vi "Main.vi"() -> ()   [LabVIEW 2017]
doc: "The myRIO Project template acquires acceleration data from the onboard accelerometer and displays the changes of acceleration values in a waveform chart."
uses:
  <vilib>/userdefined/High Color/IMAQdx.ctl
  <vilib>/Platform/TimedLoop/XDataNode/timing_clust.ctl
  <vilib>/Platform/TimedLoop/XDataNode/nitl_modes.ctl
  <vilib>/Platform/TimedLoop/XDataNode/wakeup.ctl
  <vilib>/myRIO/Common/Instrument Driver Framework/myRIO v1.0/UART/vis/myRIO v1.0 Close UART.vi
  Global 1.vi
  Outputs.vi
  Inputs.vi
  <vilib>/myRIO/Common/Instrument Driver Framework/Utilities/vis/FPGA Ref Manager.vi
  <vilib>/myRIO/Common/Instrument Driver Framework/myRIO v1.0/myRIO v1.0 Reset FPGA.vi
  <vilib>/myRIO/Common/Instrument Driver Framework/myRIO v1.0/IRQ/vis/myRIO v1.0 IRQ Info FGV.vi
  <vilib>/myRIO/Common/Instrument Driver Framework/myRIO v1.0/IRQ/vis/myRIO v1.0 Timer IRQ Info FGV.vi
  <vilib>/myRIO/Common/Instrument Driver Framework/myRIO v1.0/IRQ/vis/myRIO v1.0 ISR Agent.vi
  <vilib>/platform/TimedLoop/XDataNode/XDataNode.xnode
  <vilib>/Platform/TimedLoop/XDataNode/XDNodeRunTimeDep.lvlib
  <vilib>/myRIO/Instrument Drivers/Utilities/Utilities.lvlib
  <vilib>/vision/driver/NI_Vision_Acquisition_Software.lvlib
panel:
  out "Step":i16
  in  "Start":bool
  out "error out":errorcluster
  in  "Stop":bool
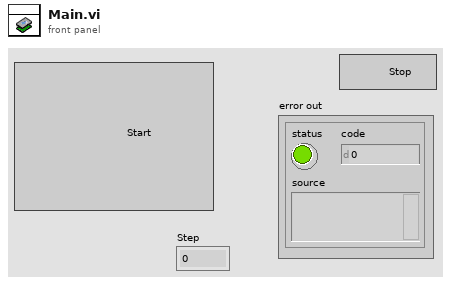
[diagram p1: front panel]
types:
  T1 = typedef "IMAQdx.ctl" = refnum<k21>
  T2 = typedef "XDNodeRunTimeDep.lvlib/timing_clust.ctl" = cluster{"Expected End [f-1]":u64, "Actual End [f-1]":u64, "Finished Late? [f-1]":bool, "Expected End [i-1]":u64, "Actual End [i-1]":u64, "Finished Late? [i-1]":bool, "Expected Start [i]":u64, "Actual Start [i]":u64, "Expected Start [f]":u64, "Actual Start [f]":u64, "Source Name":string, "Structure Name":string, "Period":i64, "Deadline":i64, "Offset":i64, "Start":i64, "Priority":i32, "Timeout":i32, "Mode":T3, "Wakeup Reason":T4, "Error":errorcluster, "Source Type":string, "Secondary Source Type":string, "Global End Time":u64, "Global Start Time":u64, "Frame Duration":u64, "Iteration Duration":u64, "Assigned CPU":i32, "I/O Scan Engine Mode":u32}
  T3 = typedef "XDNodeRunTimeDep.lvlib/nitl_modes.ctl" = enum32{"No Change", "Process missed periods, maintain original phase", "Discard missed periods, maintain original phase", "Process missed periods, ignore original phase", "Discard missed periods, ignore original phase"}
  T4 = typedef "XDNodeRunTimeDep.lvlib/wakeup.ctl" = enum32{"Normal", "Aborted", "Asynchronous wakeup", "Timing source error", "Timed loop error", "Timeout"}
  T5 = typedef "I2C.lvlib/I2C Reference.ctl" = cluster{"myRIO Reference":T6, "I2C Channels Enum":T10, "I2C Configuration":T11}
  T6 = typedef "myRIO Generic Hardware Reference.ctl" = cluster{"myRIO Model":T7, "myRIO Hardware Reference":T8}
  T7 = typedef "Hardware Version Enum.ctl" = enum16{"Unknown", "myRIO-1900", "myRIO-1950", "roboRIO", "NI ELVIS RIO CM"}
  T8 = typedef "myRIO v1.0 Reference.ctl" = cluster{"Generic FPGA Reference":T9, "Allow multiple opens":bool}
  T9 = typedef "Generic FPGA Reference.ctl" = refnum<k20>
  T10 = typedef "I2C Channels Enum.ctl" = enum16{"Not Connected", "A/I2C", "B/I2C", "I2C/I2C"}
  T11 = typedef "I2C.lvlib/I2C Configuration.ctl" = cluster{"I2C Transfer Rate":T12}
  T12 = typedef "I2C.lvlib/I2C Transfer Rate.ctl" = enum16{"Standard mode (100 kbps)", "Fast mode (400 kbps)"}
  T13 = typedef "IMAQ Image.ctl" = refnum<image>
  T14 = typedef "IMAQ GM Match Report.ctl" = cluster{"Position":cluster{"x":sgl, "y":sgl}, "Angle":sgl, "Scale":sgl, "Score":sgl, "Bounding Box":cluster{"x":sgl, "y":sgl}[], "Contrast Reversed":bool, "Occlusion %":sgl, "Template Target Curve Score":sgl, "Target Template Curve Score":sgl, "Correlation Score":sgl}
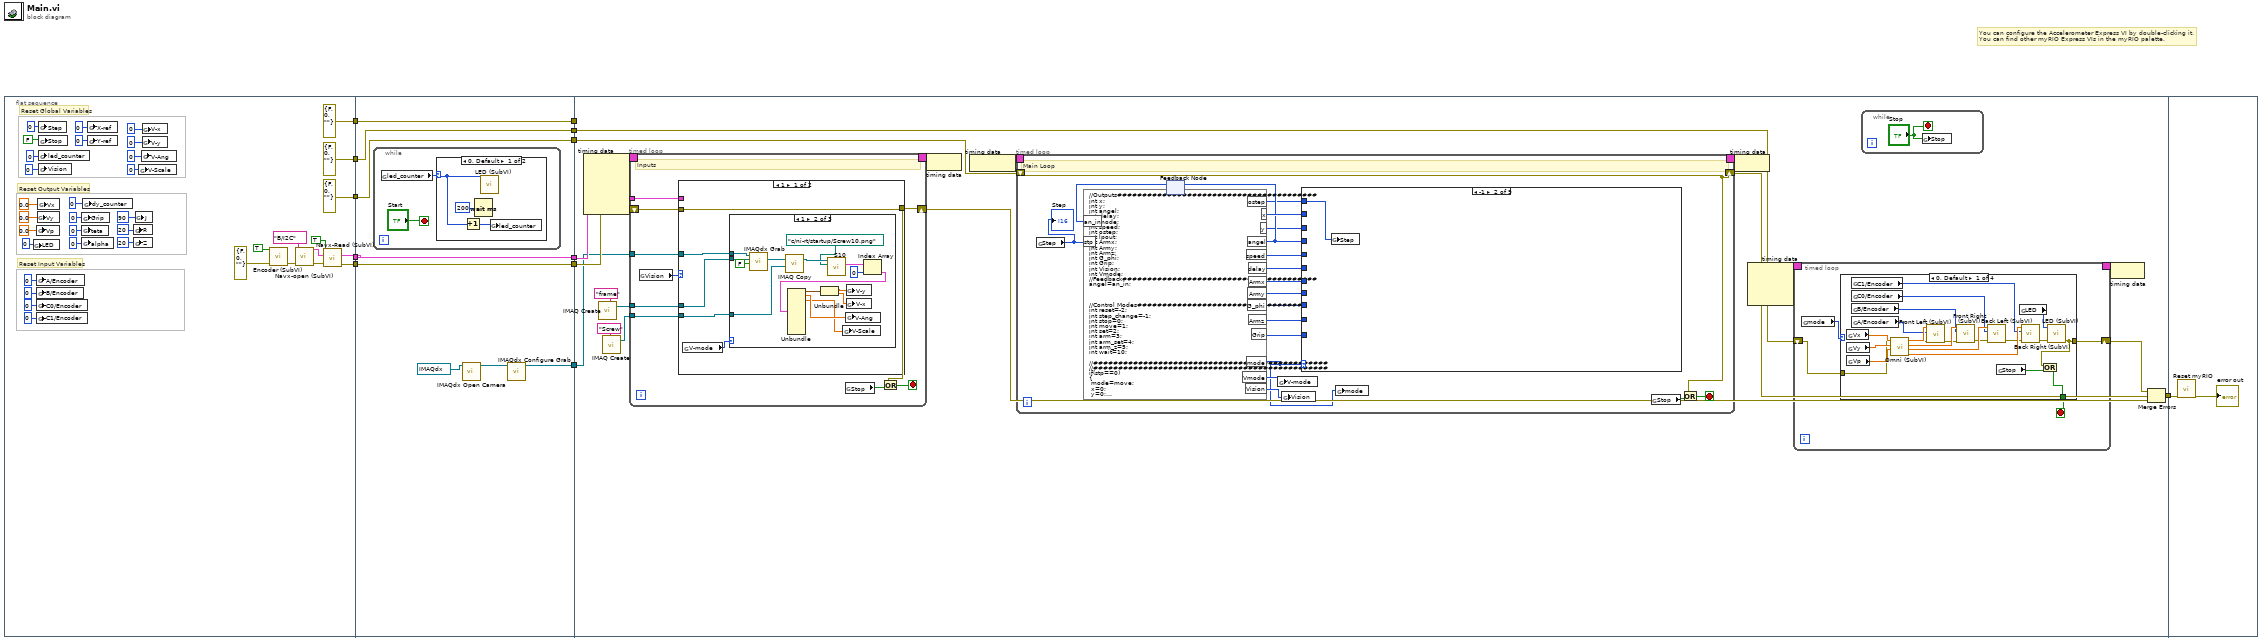
[diagram p0: block diagram]
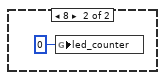
[diagram p2: hidden frame]
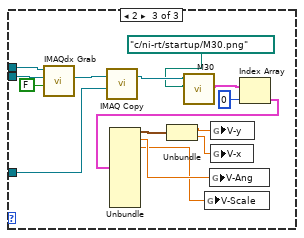
[diagram p4: hidden frame]
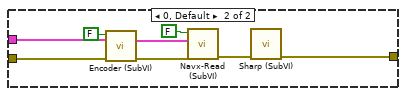
[diagram p5: hidden frame]
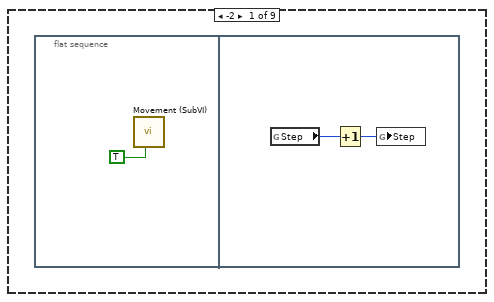
[diagram p6: hidden frame]
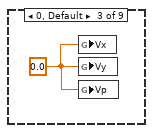
[diagram p7: hidden frame]
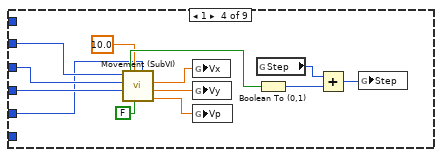
[diagram p8: hidden frame]
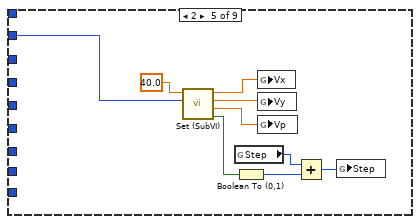
[diagram p9: hidden frame]
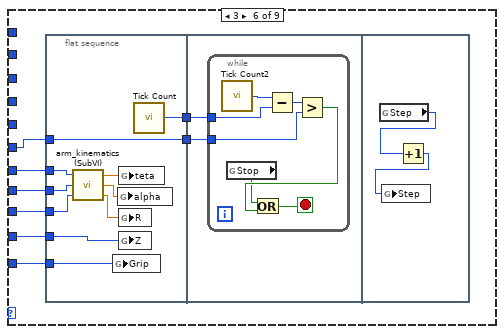
[diagram p10: hidden frame]
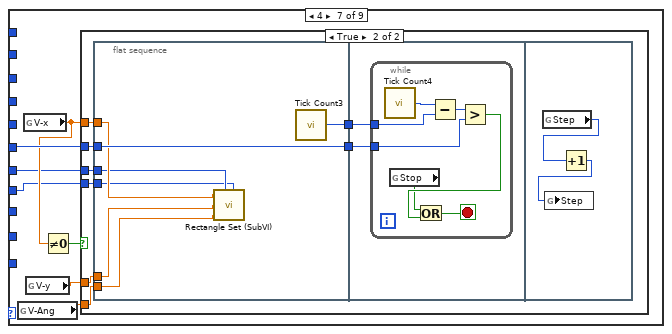
[diagram p11: hidden frame]
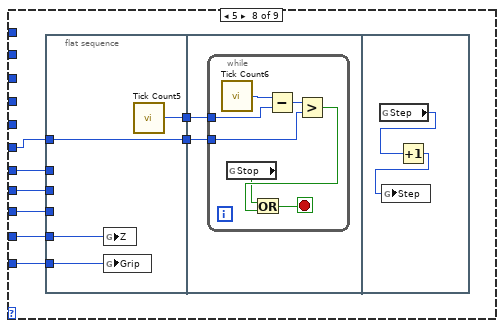
[diagram p13: hidden frame]
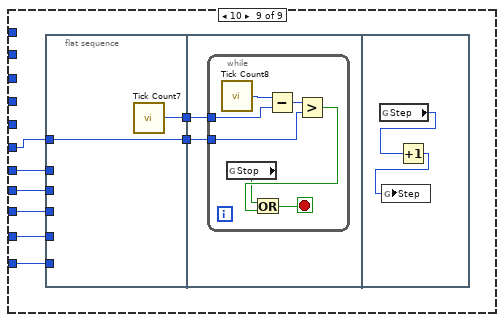
[diagram p14: hidden frame]
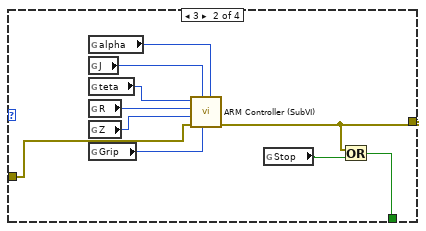
[diagram p15: hidden frame]
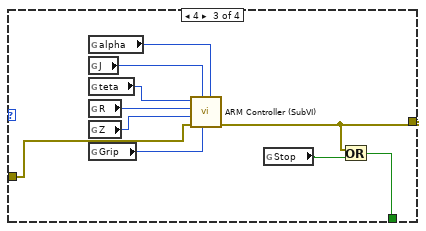
[diagram p16: hidden frame]
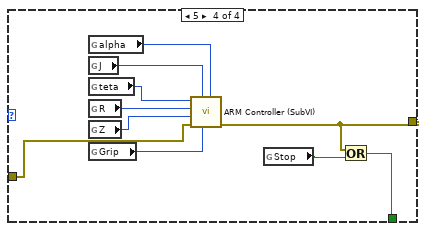
[diagram p17: hidden frame]
diagram:
  # "You can configure the Accelerometer Express VI by double-clicking it.\nYou can find other myRIO Express VIs in the myRIO palette."
  n1 = flat-sequence {
    tunnel: [w44] -> w12
    tunnel: [errorcluster {"status"=FALSE, "code"=0, "source"=""} ("error in (no error)")] -> w10
    tunnel: [errorcluster {"status"=FALSE, "code"=0, "source"=""} ("error in (no error)")] -> w8
    tunnel: [w42] -> w7
    tunnel: [errorcluster {"status"=FALSE, "code"=0, "source"=""} ("error in (no error)")] -> w4
    tunnel: w12 -> [w56]
    tunnel: [w56] -> w11
    tunnel: w10 -> [w55]
    tunnel: [w55] -> w9
    tunnel: w8 -> [w52]
    tunnel: w7 -> [w54]
    tunnel: [w54] -> w6
    tunnel: [w53] -> w5
    tunnel: w4 -> [w53]
    tunnel: [w52] -> w2
    tunnel: [w49] -> w1
    tunnel: w11 -> [w81]
    tunnel: w9 -> [_]
    tunnel: w6 -> [w74]
    tunnel: w5 -> [w73]
    tunnel: [w72] -> w3
    tunnel: w2 -> [w68]
    tunnel: w1 -> [w67]
    tunnel: w3 -> [w352]
    frame #0 {
      # "Reset Global Variables"
      # "Reset Input Variables"
      # "Reset Output Variables"
      # "Initialize"
      n2 = global write "Outputs.vi" "LED"(i8 0 ("LED")) -> ()
      n3 = global write "Outputs.vi" "Vp"(0.0 ("Vp")) -> ()
      n4 = global write "Inputs.vi" "A/Encoder"(0 ("A/Encoder")) -> ()
      n5 = global write "Inputs.vi" "B/Encoder"(0 ("B/Encoder")) -> ()
      n6 = global write "Inputs.vi" "C0/Encoder"(0 ("C0/Encoder")) -> ()
      n7 = global write "Inputs.vi" "C1/Encoder"(0 ("C1/Encoder")) -> ()
      n8 = global write "Outputs.vi" "Vy"(0.0 ("Vy")) -> ()
      n9 = global write "Outputs.vi" "Vx"(0.0 ("Vx")) -> ()
      n10 = global write "Global 1.vi" "Step"(i16 0 ("Step")) -> ()
      n11 = global write "Global 1.vi" "led_counter"(i8 0 ("Step")) -> ()
      n12 = global write "Global 1.vi" "Vision"(i8 0 ("Step")) -> ()
      n13 = global write "Global 1.vi" "Stop"(FALSE ("Stop")) -> ()
      n14 = global write "Outputs.vi" "Grip"(i16 0 ("Grip")) -> ()
      n15 = global write "Outputs.vi" "teta"(i16 0 ("teta")) -> ()
      n16 = global write "Outputs.vi" "alpha"(i16 0 ("alpha")) -> ()
      n17 = global write "Outputs.vi" "dy_counter"(i8 0 ("LED")) -> ()
      n18 = global write "Global 1.vi" "X-ref"(i64 0 ("X-ref")) -> ()
      n19 = global write "Global 1.vi" "Y-ref"(i64 0 ("Y-ref")) -> ()
      n20 = global write "Outputs.vi" "R"(i16 20 ("R")) -> ()
      n21 = global write "Outputs.vi" "Z"(i16 20 ("Z")) -> ()
      n22 = global write "Outputs.vi" "J"(i16 90 ("J")) -> ()
      n23 = global write "Global 1.vi" "V-Scale"(i64 0 ("Y-ref")) -> ()
      n24 = global write "Global 1.vi" "V-Ang"(i64 0 ("X-ref")) -> ()
      n25 = global write "Global 1.vi" "V-x"(i64 0 ("X-ref")) -> ()
      n26 = global write "Global 1.vi" "V-y"(i64 0 ("Y-ref")) -> ()
      n27 = call "Encoder (SubVI).vi"("error in (no error)"=errorcluster {"status"=FALSE, "code"=0, "source"=""}, "Reset?"=TRUE ("Reset Counter")) -> ("error out"=w26:errorcluster)  [unwired: 9 in]
      n28 = call "Navx-open (SubVI).vi"("error in (no error)"=w26, "Channel Name"=tag "B/I2C") -> ("error out"=w46:errorcluster, "I2C Ref Out"=w42:T5)  [unwired: 8 in]
      n29 = call "Navx-Read (SubVI).vi"("error in (no error)"=w46, "I2C Ref Out"=w42, "Reset"=TRUE) -> ("error out"=w44:errorcluster)  [unwired: 7 in, 1 out]
    }
    frame #1 {
      n30 = while {
        stop <- "Start" stop-if-true
        n31 = global read "Global 1.vi" "led_counter"() -> (w57:i8)
        n32 = case shown="0, Default" w57 {
          selector: w57 -> [w59 _]
          frame 0, Default {
            n33 = Increment(x=w59) -> (x+1=w61:i8)
            n34 = Wait (ms)(milliseconds to wait=u32 200) -> ()  [unwired: 1 out]
            n35 = call "LED (SubVI).vi"("LED"=w59) -> ()  [unwired: 10 in, 1 out]
            n36 = global write "Global 1.vi" "led_counter"(w61) -> ()
          }
          frame 8 {
            n37 = global write "Global 1.vi" "led_counter"(i8 0 ("led_counter")) -> ()
          }
        }
      }
      n38 = call <vilib>:"IMAQdx Open Camera.vi"("Session In"=T1 "cam0") -> ("Session Out"=w50:T1)  [unwired: 9 in, 1 out]
      n39 = call <vilib>:"IMAQdx Configure Grab.vi"("Session In"=w50) -> ("Session Out"=w49:T1)  [unwired: 9 in, 1 out]
    }
    frame #2 {
      n40 = node-c288() -> (w76:T2)  [unwired: 5 in]
      n41 = call "IMAQ Create"("Image Name"="frame") -> ("New Image"=w64:T13)  [unwired: 4 in, 1 out]
      n42 = call "IMAQ Create"("Image Name"="Screw") -> ("New Image"=w63:T13)  [unwired: 4 in, 1 out]
      n43 = timed-loop {
        shift-right: [w86] -> w71
        shift-left: w81 -> [w90]
        timing: w76 -> [_]
        timing-out: [_] -> w75
        tunnel: w74 -> [w88]
        tunnel: w67 -> [w84]
        tunnel: w64 -> [w83]
        tunnel: w63 -> [w82]
        stop <- w89 stop-if-true
        # "Inputs"
        n44 = global read "Global 1.vi" "Vision"() -> (w85:i16)
        n45 = case shown="1" w85 {
          tunnel: w90 -> [w92 w132]
          tunnel: w88 -> [_ w129]
          tunnel: [w92 w127] -> w86
          tunnel: w84 -> [w95 _]
          tunnel: w83 -> [w94 _]
          tunnel: w82 -> [w93 _]
          frame 1 {
            n46 = global read "Global 1.vi" "V-mode"() -> (w91:i16)
            n47 = case shown="1" w91 {
              tunnel: w94 -> [_ w108 w124]
              tunnel: w93 -> [_ w107 w123]
              tunnel: w95 -> [_ w97 w115]
              frame 0, Default {
              }
              frame 1 {
                n48 = call <vilib>:"IMAQdx Grab.vi"("Wait for Next Buffer? (Yes)"=FALSE, "Image In"=w108, "Session In"=w97) -> ("Image Out"=w110:T13)  [unwired: 5 in, 3 out]
                n49 = call "IMAQ Copy"("Image Dst"=w107, "Image Src"=w110) -> ("Image Dst Out"=w109:T13)  [unwired: 4 in, 1 out]
                n50 = call "S10.vi"("Template File Path (Geometric Matching 1)"=path "c:/ni-rt/startup/Screw10.png", "Image In"=w109) -> ("Matches (Geometric Matching 1)"=w105:T14[])  [unwired: 5 in, 2 out]
                n51 = Index Array(array=w105, index=0) -> (element=w103:T14)
                n52 = Unbundle(w103) -> ("Position"=w102:cluster{"x":sgl, "y":sgl}, "Angle"=w99:sgl, "Scale"=w98:sgl)  [unwired: 7 out]
                n53 = Unbundle(w102) -> ("x"=w101:sgl, "y"=w100:sgl)
                n54 = global write "Global 1.vi" "V-Scale"(w98) -> ()
                n55 = global write "Global 1.vi" "V-Ang"(w99) -> ()
                n56 = global write "Global 1.vi" "V-y"(w101) -> ()
                n57 = global write "Global 1.vi" "V-x"(w100) -> ()
              }
              frame 2 {
                n58 = call <vilib>:"IMAQdx Grab.vi"("Wait for Next Buffer? (Yes)"=FALSE, "Image In"=w124, "Session In"=w115) -> ("Image Out"=w125:T13)  [unwired: 5 in, 3 out]
                n59 = call "IMAQ Copy"("Image Dst"=w123, "Image Src"=w125) -> ("Image Dst Out"=w113:T13)  [unwired: 4 in, 1 out]
                n60 = call "M30.vi"("Template File Path (Geometric Matching 1)"=path "c:/ni-rt/startup/M30.png", "Image In"=w113) -> ("Matches (Geometric Matching 1)"=w114:T14[])  [unwired: 3 in, 2 out]
                n61 = Index Array(array=w114, index=0) -> (element=w121:T14)
                n62 = Unbundle(w121) -> ("Position"=w120:cluster{"x":sgl, "y":sgl}, "Angle"=w117:sgl, "Scale"=w116:sgl)  [unwired: 7 out]
                n63 = Unbundle(w120) -> ("x"=w119:sgl, "y"=w118:sgl)
                n64 = global write "Global 1.vi" "V-Scale"(w116) -> ()
                n65 = global write "Global 1.vi" "V-Ang"(w117) -> ()
                n66 = global write "Global 1.vi" "V-y"(w119) -> ()
                n67 = global write "Global 1.vi" "V-x"(w118) -> ()
              }
            }
          }
          frame 0, Default {
            n68 = call "Encoder (SubVI).vi"("error in (no error)"=w132, "Reset?"=FALSE ("Boolean")) -> ("error out"=w130:errorcluster)  [unwired: 9 in]
            n69 = call "Navx-Read (SubVI).vi"("error in (no error)"=w130, "I2C Ref Out"=w129, "Reset"=FALSE) -> ("error out"=w128:errorcluster)  [unwired: 7 in, 1 out]
            n70 = call "Sharp (SubVI).vi"("error in (no error)"=w128) -> ("error out"=w127:errorcluster)  [unwired: 10 in]
          }
        }
        n71 = global read "Global 1.vi" "Stop"() -> (w87:bool)
        n72 = Or(x=w86, y=w87) -> (x .or. y?=w89:bool)
      }
      n73 = node-c288(w75) -> ()
      n74 = node-c288() -> (w78:T2)
      n75 = timed-loop {
        shift-right: [w154] -> w70
        shift-left: w68 -> [w154]
        timing: w78 -> [_]
        timing-out: [_] -> w77
        stop <- w155 stop-if-true
        # "Main Loop"
        n76 = global read "Global 1.vi" "Step"() -> (w147:i16)
        "Step" <- w147
        n77 = feedback #1() -> (w151:i32)  [unwired: 1 in]
        n78 = formula code="//Outputs########################################\nint x;\nint y;\nint angel;\nint delay;\nint mode;\nint speed;\nint ostep;\nint lpout;\nint Armx;\nint Army;\nint Armz;\nint G_phi;\nint Grip;\nint Vision;\nint Vmode;\n//Feedback#######################################\nangel=an_in;\n\n\n\n//Control Modes##################################\nint reset=-2;\nint step_change=-1; \nint stop=0;\nint move=1;\nint set=2;\nint arm=3;\nint arm_set=4;\nint arm_z=5;\nint wait=10;\n\n//###############################################\n//###############################################\nif(stp==0)\n{\n\tmode=move;\n\tx=0;\n\ty=0;\n\tangel=0;\n\tspeed=50;\n}\nif(stp==1)\n{\n\tmode=arm;\n\tArmx=75;\n\tArmy=0;\n\tArmz=180;\n\tdelay=4000;\n\t\n}\nif(stp==2)\n{\n\tmode=step_change;\n\tostep=5;\n}\nif(stp==3)\n{\n\tmode=move;\n\tx=0;\n\ty=0;\n\tangel=-90;\n\tspeed=80;\n}\nif(stp==4)\n{\n\tmode=move;\n\tx=800;\n\ty=0;\n\tangel=0;\n\tspeed=80;\n}\nif(stp==5)\n{\n\tmode=set;\n\tx=3;\n\tspeed=50;\n}\nif(stp==6)\n{\n\tmode=reset;\n}\n\nif(stp==7)\n{\n\tmode=arm;\n\tArmx=75;\n\tArmy=0;\n\tArmz=280;\n\tdelay=4000;\n}\nif(stp==8)\n{\n\tVision=1;\n\tVmode=1;\n\tmode=wait;\n\tdelay=1500;\n}\nif(stp==9)\n{\n\tVision=1;\n\tVmode=1;\n\tmode=arm_set;\n\tArmx=75;\n\tArmy=0;\n\tdelay=4000;\n}\nif(stp==10)\n{\n\tVision=0;\n\tmode=wait;\n\tdelay=1000;\n}\nif(stp==11)\n{\n\tVision=0;\n\tmode=arm_z;\n\tArmz=100;\n\tGrip=0;\n\tdelay=3000;\n}\nif(stp==12)\n{\n\tmode=arm_z;\n\tArmz=100;\n\tGrip=1;\n\tdelay=1000;\n}\nif(stp==13)\n{\n\tmode=arm_z;\n\tArmz=200;\n\tGrip=1;\n\tdelay=1000;\n}\nif(stp==14)\n{\n\tmode=arm;\n\tArmx=75;\n\tArmy=0;\n\tArmz=200;\n\tGrip=1;\n\tdelay=4000;\n}\n\n\n\nif(stp==15)\n{\n\tmode=stop;\n}"("stp"=w147, "an_in"=w151) -> ("x"=w153:i32, "y"=w148:i32, "mode"=w137:i32, "angel"=w150:i32, "delay"=w152:i32, "speed"=w149:i32, "ostep"=w145:i32, "Armx"=w143:i32, "Army"=w142:i32, "Armz"=w141:i32, "G_phi"=w144:i32, "Grip"=w140:i32, "Vision"=w139:i32, "Vmode"=w138:i32)
        n79 = feedback-in #1(w150) -> ()
        n80 = global write "Global 1.vi" "V-mode"(w138) -> ()
        n81 = global write "Global 1.vi" "Vision"(w139) -> ()
        n82 = case shown="-1" w137 {
          tunnel: w153 -> [_ _ _ w167 w182 _ _ _ _]
          tunnel: w148 -> [_ _ _ w166 _ _ _ _ _]
          tunnel: w150 -> [_ _ _ w165 _ _ _ _ _]
          tunnel: w152 -> [_ _ _ _ _ w189 w218 w251 w274]
          tunnel: w149 -> [_ _ _ w164 _ _ _ _ _]
          tunnel: w145 -> [_ w159 _ _ _ _ _ _ _]
          tunnel: w144 -> [_ _ _ _ _ w185 _ w247 w270]
          tunnel: w143 -> [_ _ _ _ _ w187 w213 w249 w272]
          tunnel: w142 -> [_ _ _ _ _ w186 w212 w248 w271]
          tunnel: w141 -> [_ _ _ _ _ w184 _ w246 w269]
          tunnel: w140 -> [_ _ _ _ _ w183 _ w245 w268]
          frame -2 {
            n83 = flat-sequence {
              frame #0 {
                n84 = call "Movement (SubVI).vi"("Reset"=TRUE) -> ()  [unwired: 6 in, 4 out]
              }
              frame #1 {
                n85 = global read "Global 1.vi" "Step"() -> (w158:i16)
                n86 = Increment(x=w158) -> (x+1=w157:i16)
                n87 = global write "Global 1.vi" "Step"(w157) -> ()
              }
            }
          }
          frame -1 {
            n88 = global write "Global 1.vi" "Step"(w159) -> ()
          }
          frame 0, Default {
            w160 = 0.0 ("Vy")
            n89 = global write "Outputs.vi" "Vx"(w160) -> ()
            n90 = global write "Outputs.vi" "Vy"(w160) -> ()
            n91 = global write "Outputs.vi" "Vp"(w160) -> ()
          }
          frame 1 {
            n92 = call "Movement (SubVI).vi"("Speed"=w164, "Reset"=FALSE, "Acc"=10.0, "Goal P"=w165, "Goal Y"=w166, "Goal X"=w167) -> ("Vp"=w169:dbl, "Vy"=w170:dbl, "Vx"=w171:dbl, "Reach?"=w172:bool)  [unwired: 1 in]
            n93 = global write "Outputs.vi" "Vx"(w171) -> ()
            n94 = global write "Outputs.vi" "Vy"(w170) -> ()
            n95 = global write "Outputs.vi" "Vp"(w169) -> ()
            n96 = global read "Global 1.vi" "Step"() -> (w161:i16)
            n97 = Boolean To (0,1)(Boolean=w172) -> (0, 1=w173:i16)
            n98 = Add(x=w161, y=w173) -> (x+y=w162:i16)
            n99 = global write "Global 1.vi" "Step"(w162) -> ()
          }
          frame 2 {
            n100 = call "Set (SubVI).vi"("Mode"=w182, "speed"=40.0) -> ("Reach?"=w174:bool, "Vp"=w178:dbl, "Vy"=w179:dbl, "Vx"=w180:dbl)  [unwired: 4 in]
            n101 = global read "Global 1.vi" "Step"() -> (w175:i16)
            n102 = Boolean To (0,1)(Boolean=w174) -> (0, 1=w177:i16)
            n103 = global write "Outputs.vi" "Vx"(w180) -> ()
            n104 = global write "Outputs.vi" "Vy"(w179) -> ()
            n105 = global write "Outputs.vi" "Vp"(w178) -> ()
            n106 = Add(x=w175, y=w177) -> (x+y=w176:i16)
            n107 = global write "Global 1.vi" "Step"(w176) -> ()
          }
          frame 3 {
            n108 = flat-sequence {
              tunnel: [w200] -> w190
              tunnel: w189 -> [w196]
              tunnel: [w196] -> w188
              tunnel: w187 -> [w195]
              tunnel: w186 -> [w194]
              tunnel: w185 -> [w193]
              tunnel: w184 -> [w192]
              tunnel: w183 -> [w191]
              tunnel: w190 -> [w202]
              tunnel: w188 -> [w201]
              frame #0 {
                n109 = call "arm_kinematics (SubVI).vi"("alpha"=w193, "y"=w194, "x"=w195) -> ("R"=w197:dbl, "alpha"=w198:dbl, "teta"=w199:dbl)
                n110 = global write "Outputs.vi" "Grip"(w191) -> ()
                n111 = global write "Outputs.vi" "alpha"(w198) -> ()
                n112 = global write "Outputs.vi" "teta"(w199) -> ()
                n113 = global write "Outputs.vi" "R"(w197) -> ()
                n114 = global write "Outputs.vi" "Z"(w192) -> ()
                n115 = call "Tick Count"() -> ("Tick Count(mSec)"=w200:u32)
              }
              frame #1 {
                n116 = while {
                  tunnel: w202 -> [w208]
                  tunnel: w201 -> [w203]
                  stop <- w205 stop-if-true
                  n117 = call "Tick Count2"() -> ("Tick Count(mSec)"=w209:u32)
                  n118 = global read "Global 1.vi" "Stop"() -> (w204:bool)
                  n119 = Subtract(x=w209, y=w208) -> (x-y=w207:u32)
                  n120 = Greater?(x=w207, y=w203) -> (0:w206:bool)
                  n121 = Or(x=w204, y=w206) -> (x .or. y?=w205:bool)
                }
              }
              frame #2 {
                n122 = global read "Global 1.vi" "Step"() -> (w210:i16)
                n123 = Increment(x=w210) -> (x+1=w211:i16)
                n124 = global write "Global 1.vi" "Step"(w211) -> ()
              }
            }
          }
          frame 4 {
            n125 = global read "Global 1.vi" "V-Ang"() -> (w214:sgl)
            n126 = global read "Global 1.vi" "V-x"() -> (w215:sgl)
            n127 = global read "Global 1.vi" "V-y"() -> (w217:sgl)
            n128 = Not Equal To 0?(x=w215) -> (x != 0?=w216:bool)
            n129 = case shown="True" w216 {
              tunnel: w218 -> [_ w224]
              tunnel: w217 -> [_ w223]
              tunnel: w215 -> [_ w222]
              tunnel: w214 -> [_ w221]
              tunnel: w213 -> [_ w220]
              tunnel: w212 -> [_ w219]
              frame False {
              }
              frame True {
                n130 = flat-sequence {
                  tunnel: [w233] -> w226
                  tunnel: w224 -> [w232]
                  tunnel: [w232] -> w225
                  tunnel: w223 -> [w230]
                  tunnel: w222 -> [w231]
                  tunnel: w221 -> [w229]
                  tunnel: w220 -> [w228]
                  tunnel: w219 -> [w227]
                  tunnel: w226 -> [w235]
                  tunnel: w225 -> [w234]
                  frame #0 {
                    n131 = call "Rectangle Set (SubVI).vi"("x"=w231, "x in"=w228, "y"=w230, "alpha"=w229, "y in"=w227) -> ()  [unwired: 6 in]
                    n132 = call "Tick Count3"() -> ("Tick Count(mSec)"=w233:u32)
                  }
                  frame #1 {
                    n133 = while {
                      tunnel: w235 -> [w241]
                      tunnel: w234 -> [w236]
                      stop <- w238 stop-if-true
                      n134 = call "Tick Count4"() -> ("Tick Count(mSec)"=w242:u32)
                      n135 = global read "Global 1.vi" "Stop"() -> (w237:bool)
                      n136 = Subtract(x=w242, y=w241) -> (x-y=w240:u32)
                      n137 = Greater?(x=w240, y=w236) -> (0:w239:bool)
                      n138 = Or(x=w237, y=w239) -> (x .or. y?=w238:bool)
                    }
                  }
                  frame #2 {
                    n139 = global read "Global 1.vi" "Step"() -> (w243:i16)
                    n140 = Increment(x=w243) -> (x+1=w244:i16)
                    n141 = global write "Global 1.vi" "Step"(w244) -> ()
                  }
                }
              }
            }
          }
          frame 5 {
            n142 = flat-sequence {
              tunnel: [w256] -> w252
              tunnel: w251 -> [w255]
              tunnel: [w255] -> w250
              tunnel: w249 -> [_]
              tunnel: w248 -> [_]
              tunnel: w247 -> [_]
              tunnel: w246 -> [w254]
              tunnel: w245 -> [w253]
              tunnel: w252 -> [w258]
              tunnel: w250 -> [w257]
              frame #0 {
                n143 = global write "Outputs.vi" "Z"(w254) -> ()
                n144 = global write "Outputs.vi" "Grip"(w253) -> ()
                n145 = call "Tick Count5"() -> ("Tick Count(mSec)"=w256:u32)
              }
              frame #1 {
                n146 = while {
                  tunnel: w258 -> [w264]
                  tunnel: w257 -> [w259]
                  stop <- w261 stop-if-true
                  n147 = call "Tick Count6"() -> ("Tick Count(mSec)"=w265:u32)
                  n148 = global read "Global 1.vi" "Stop"() -> (w260:bool)
                  n149 = Subtract(x=w265, y=w264) -> (x-y=w263:u32)
                  n150 = Greater?(x=w263, y=w259) -> (0:w262:bool)
                  n151 = Or(x=w260, y=w262) -> (x .or. y?=w261:bool)
                }
              }
              frame #2 {
                n152 = global read "Global 1.vi" "Step"() -> (w266:i16)
                n153 = Increment(x=w266) -> (x+1=w267:i16)
                n154 = global write "Global 1.vi" "Step"(w267) -> ()
              }
            }
          }
          frame 10 {
            n155 = flat-sequence {
              tunnel: [w277] -> w275
              tunnel: w274 -> [w276]
              tunnel: [w276] -> w273
              tunnel: w272 -> [_]
              tunnel: w271 -> [_]
              tunnel: w270 -> [_]
              tunnel: w269 -> [_]
              tunnel: w268 -> [_]
              tunnel: w275 -> [w279]
              tunnel: w273 -> [w278]
              frame #0 {
                n156 = call "Tick Count7"() -> ("Tick Count(mSec)"=w277:u32)
              }
              frame #1 {
                n157 = while {
                  tunnel: w279 -> [w285]
                  tunnel: w278 -> [w280]
                  stop <- w282 stop-if-true
                  n158 = call "Tick Count8"() -> ("Tick Count(mSec)"=w286:u32)
                  n159 = global read "Global 1.vi" "Stop"() -> (w281:bool)
                  n160 = Subtract(x=w286, y=w285) -> (x-y=w284:u32)
                  n161 = Greater?(x=w284, y=w280) -> (0:w283:bool)
                  n162 = Or(x=w281, y=w283) -> (x .or. y?=w282:bool)
                }
              }
              frame #2 {
                n163 = global read "Global 1.vi" "Step"() -> (w287:i16)
                n164 = Increment(x=w287) -> (x+1=w288:i16)
                n165 = global write "Global 1.vi" "Step"(w288) -> ()
              }
            }
          }
        }
        n166 = global write "Global 1.vi" "mode"(w137) -> ()
        n167 = global read "Global 1.vi" "Stop"() -> (w146:bool)
        n168 = Or(x=w154, y=w146) -> (x .or. y?=w155:bool)
      }
      n169 = node-c288(w77) -> ()
      n170 = node-c288() -> (w80:T2)  [unwired: 3 in]
      n171 = timed-loop {
        timing: w80 -> [_]
        timing-out: [_] -> w79
        shift-right: [w294] -> w69
        shift-left: w73 -> [w295]
        stop <- w296 stop-if-true
        n172 = global read "Global 1.vi" "mode"() -> (w293:i16)
        n173 = case shown="0, Default" w293 {
          tunnel: [w313 w317 w327 w337] -> w296
          tunnel: w295 -> [w305 w319 w329 w339]
          tunnel: [w298 w318 w328 w338] -> w294
          frame 0, Default {
            n174 = global read "Outputs.vi" "Vx"() -> (w312:dbl)
            n175 = global read "Outputs.vi" "Vy"() -> (w315:dbl)
            n176 = global read "Outputs.vi" "Vp"() -> (w314:dbl)
            n177 = global read "Inputs.vi" "C1/Encoder"() -> (w304:i32)
            n178 = global read "Inputs.vi" "C0/Encoder"() -> (w303:i32)
            n179 = global read "Inputs.vi" "B/Encoder"() -> (w302:i32)
            n180 = global read "Inputs.vi" "A/Encoder"() -> (w301:i32)
            n181 = call "Omni (SubVI).vi"("Vp"=w314, "Vy"=w315, "Vx"=w312) -> ("Back_Right"=w310:dbl, "Back_Left"=w316:dbl, "Front_Right"=w311:dbl, "Front_Left"=w308:dbl)  [unwired: 4 in]
            n182 = call "Front Left (SubVI).vi"("setpoint"=w308, "Counter Value"=w301, "error in"=w305) -> ("error out"=w309:errorcluster)  [unwired: 6 in, 1 out]
            n183 = call "Front Right (SubVI).vi"("error in"=w309, "Counter Value"=w302, "setpoint"=w311) -> ("error out"=w307:errorcluster)  [unwired: 7 in, 1 out]
            n184 = call "Back Left (SubVI).vi"("error in"=w307, "Counter Value"=w303, "setpoint"=w316) -> ("error out"=w306:errorcluster)  [unwired: 7 in, 1 out]
            n185 = global read "Global 1.vi" "Stop"() -> (w300:bool)
            n186 = global read "Outputs.vi" "LED"() -> (w297:i8)
            n187 = call "Back Right (SubVI).vi"("error in"=w306, "Counter Value"=w304, "setpoint"=w310) -> ("error out"=w299:errorcluster)  [unwired: 7 in, 1 out]
            n188 = call "LED (SubVI).vi"("error in (no error)"=w299, "LED"=w297) -> ("error out"=w298:errorcluster)  [unwired: 9 in]
            n189 = Or(x=w298, y=w300) -> (x .or. y?=w313:bool)
          }
          frame 3 {
            n190 = global read "Outputs.vi" "alpha"() -> (w321:i16)
            n191 = global read "Outputs.vi" "J"() -> (w322:i16)
            n192 = global read "Outputs.vi" "teta"() -> (w326:i16)
            n193 = global read "Outputs.vi" "R"() -> (w325:i16)
            n194 = global read "Outputs.vi" "Z"() -> (w324:i16)
            n195 = global read "Outputs.vi" "Grip"() -> (w323:i16)
            n196 = call "ARM Controller (SubVI).vi"("alpha"=w321, "Grip"=w323, "J"=w322, "error in (no error)"=w319, "Z"=w324, "R"=w325, "teta"=w326) -> ("error out"=w318:errorcluster)  [unwired: 4 in]
            n197 = global read "Global 1.vi" "Stop"() -> (w320:bool)
            n198 = Or(x=w318, y=w320) -> (x .or. y?=w317:bool)
          }
          frame 4 {
            n199 = global read "Outputs.vi" "alpha"() -> (w331:i16)
            n200 = global read "Outputs.vi" "J"() -> (w332:i16)
            n201 = global read "Outputs.vi" "teta"() -> (w336:i16)
            n202 = global read "Outputs.vi" "R"() -> (w335:i16)
            n203 = global read "Outputs.vi" "Z"() -> (w334:i16)
            n204 = global read "Outputs.vi" "Grip"() -> (w333:i16)
            n205 = call "ARM Controller (SubVI).vi"("alpha"=w331, "Grip"=w333, "J"=w332, "error in (no error)"=w329, "Z"=w334, "R"=w335, "teta"=w336) -> ("error out"=w328:errorcluster)  [unwired: 4 in]
            n206 = global read "Global 1.vi" "Stop"() -> (w330:bool)
            n207 = Or(x=w328, y=w330) -> (x .or. y?=w327:bool)
          }
          frame 5 {
            n208 = global read "Outputs.vi" "alpha"() -> (w341:i16)
            n209 = global read "Outputs.vi" "J"() -> (w342:i16)
            n210 = global read "Outputs.vi" "teta"() -> (w346:i16)
            n211 = global read "Outputs.vi" "R"() -> (w345:i16)
            n212 = global read "Outputs.vi" "Z"() -> (w344:i16)
            n213 = global read "Outputs.vi" "Grip"() -> (w343:i16)
            n214 = call "ARM Controller (SubVI).vi"("alpha"=w341, "Grip"=w343, "J"=w342, "error in (no error)"=w339, "Z"=w344, "R"=w345, "teta"=w346) -> ("error out"=w338:errorcluster)  [unwired: 4 in]
            n215 = global read "Global 1.vi" "Stop"() -> (w340:bool)
            n216 = Or(x=w338, y=w340) -> (x .or. y?=w337:bool)
          }
        }
      }
      n217 = while {
        stop <- "Stop" stop-if-true
        n218 = global write "Global 1.vi" "Stop"("Stop") -> ()
      }
      n219 = node-c288(w79) -> ()
      n220 = Merge Errors(w69, w70, w71) -> (w72:errorcluster)
    }
    frame #3 {
      # "Close"
      n221 = call <vilib>:"Reset myRIO.vi"("error in (no error)"=w352) -> ("error out"=→"error out":errorcluster)  [unwired: 10 in]
    }
  }
